vi "main.vi"() -> ()   [LabVIEW 2022 SP3]
panel:
  out "return value":i32[](array[numeric])
  out "error out":errorcluster
  in  "error in":errorcluster
  out "Bool Array":bool[](array[boolean])
  # "SW1"
  # "SW2"
  # "SW3"
  # "SW4"
  # "SW5"
  # "SW6"
  # "SW7"
  # "SW8"
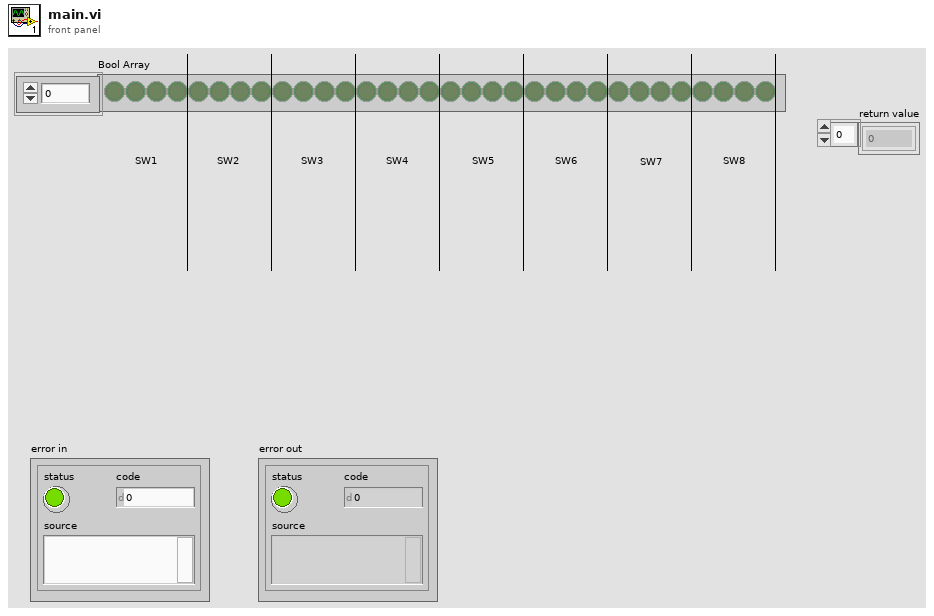
[diagram p1: front panel]
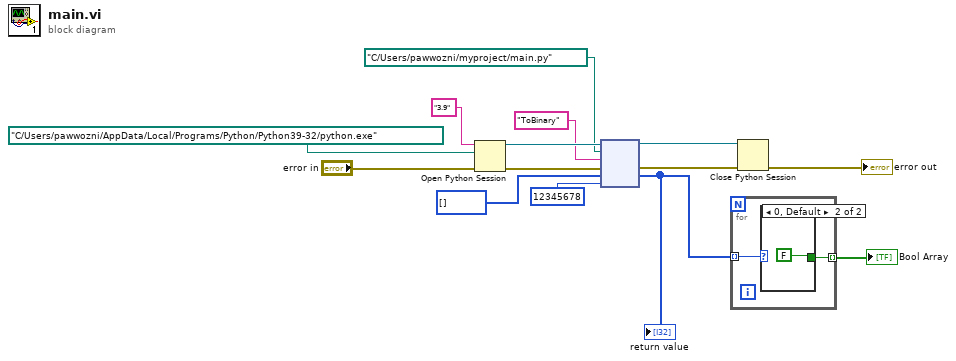
[diagram p0: block diagram]
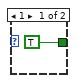
[diagram p2: hidden frame]
diagram:
  n1 = Open Python Session(python version="3.9" ("Python version"), python path=path "C:/Users/pawwozni/AppData/Local/Programs/Python/Python39-32/python.exe" ("Python path"), 3:"error in") -> (session out=w10:refnum<k35>, error out=w9:errorcluster)
  n2 = node(w10, path "C:/Users/pawwozni/myproject/main.py" ("Python path"), "ToBinary" ("function name"), w9, i32[] [], u32 12345678) -> (w5:refnum<k35>, w4:errorcluster, w3:i32[])  [unwired: 1 in, 2 out]
  "return value" <- w3
  n3 = for {
    tunnel: w3 -> [w16] mode=indexing
    tunnel: [w15] -> w2 mode=indexing
    n4 = case shown="0, Default" w16 {
      tunnel: [TRUE FALSE] -> w15
      frame 1 {
      }
      frame 0, Default {
      }
    }
  }
  "Bool Array" <- w2
  n5 = Close Python Session(session in=w5, error in=w4) -> (11:→"error out":errorcluster)
